vi "Square_Pyramid_Vol_Calc.vi"() -> ()   [LabVIEW 2025]
panel:
  out "Volume":dbl
  in  "Base edge":dbl
  in  "Height":dbl
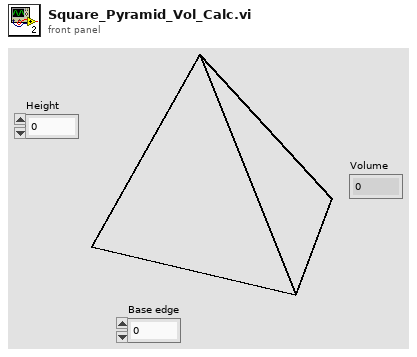
[diagram p1: front panel]
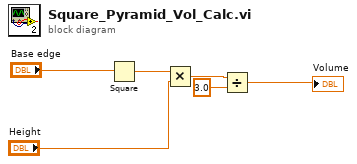
[diagram p0: block diagram]
diagram:
  n1 = Square(x="Base edge") -> (x^2=w6:dbl)
  n2 = Multiply(x=w6, y="Height") -> (x*y=w3:dbl)
  n3 = Divide(x=w3, y=3.0) -> (x/y=→"Volume":dbl)
